vi "is_in_range.vi"(8 "error in (no error)":errorcluster caption="错误输入（无错误）", 11 "OneMotion 输入":refnum<class "OneMotion.lvclass">) -> (0 "error out":errorcluster caption="错误输出", 3 "OneMotion 输出":refnum<class "OneMotion.lvclass">)   [LabVIEW 2016, in "MotionControl.lvlib" / "OneMotion.lvclass"]
uses:
  <userlib>/MotionControl/OneMotion/OneMotion.lvclass
  <userlib>/MotionControl/OneMotion/OneMotion.lvclass/OneMotion.ctl
panel:
  out "is in range?":bool
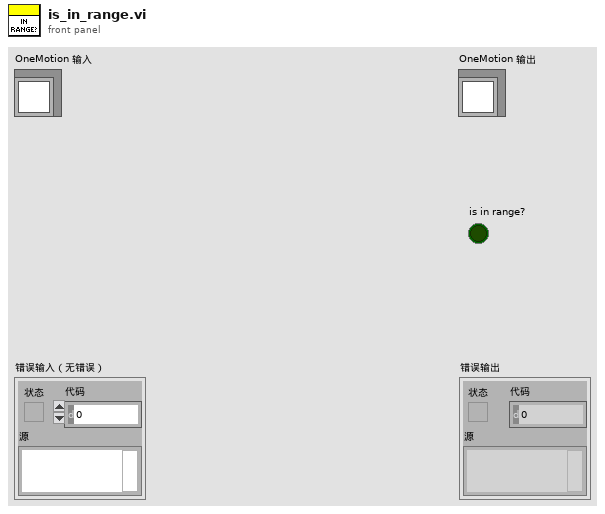
[diagram p1: front panel]
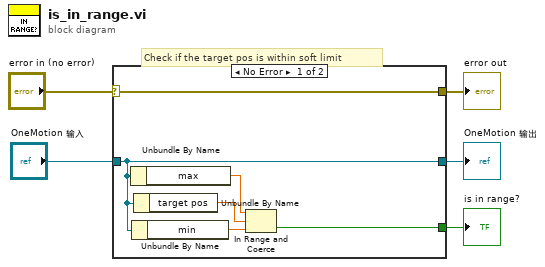
[diagram p0: block diagram]
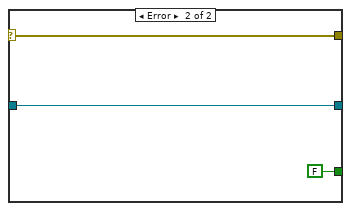
[diagram p2: hidden frame]
diagram:
  # "Check if the target pos is within soft limit"
  n1 = case shown="No Error" "error in (no error)" {
    selector: "error in (no error)" -> [w9 w14]
    tunnel: [w9 w14] -> w4
    tunnel: [w8 w13] -> w2
    tunnel: "OneMotion 输入" -> [w8 w13]
    tunnel: [w10 FALSE] -> w1
    frame No Error {
      n2 = Unbundle By Name(w8) -> ("max"=w7:dbl)
      n3 = Unbundle By Name(w8) -> ("min"=w6:dbl)
      n4 = Unbundle By Name(w8) -> ("target pos"=w11:dbl)
      n5 = In Range and Coerce(upper limit=w7, x=w11, lower limit=w6) -> (In Range?=w10:bool)  [unwired: 1 out]
    }
    frame Error {
    }
  }
  "error out" <- w4
  "OneMotion 输出" <- w2
  "is in range?" <- w1
